vi "GeoData.vi"() -> ()   [LabVIEW 2017] (continued)
H1\n17261\t42055\tSouth mountain\tPA\tFranklin County\tH1\n17225\t42055\tGreencastle\tPA\tFranklin County\tH1\n17257\t42055\tShippensburg\tPA\tFranklin County\tH1\n17263\t42055\tState line\tPA\tFranklin County\tH1\n17251\t42055\tRoxbury\tPA\tFranklin County\tH1\n17211\t42057\tArtemas\tPA\tFulton County\tH1\n17238\t42057\tNeedmore\tPA\tFulton County\tH1\n17228\t42057\tHarrisonville\tPA\tFulton County\tH1\n17264\t42057\tThree springs\tPA\tFulton County\tH1\n17236\t42057\tMercersburg\tPA\tFulton County\tH1\n15533\t42057\tBreezewood\tPA\tFulton County\tH1\n17224\t42057\tFort loudon\tPA\tFulton County\tH1\n16689\t42057\tWaterfall\tPA\tFulton County\tH1\n16691\t42057\tWells tannery\tPA\tFulton County\tH1\n17255\t42057\tShade gap\tPA\tFulton County\tH1\n15536\t42057\tCrystal spring\tPA\tFulton County\tH1\n17233\t42057\tMc connellsburg\tPA\tFulton County\tH1\n17267\t42057\tWarfordsburg\tPA\tFulton County\tH1\n16674\t42057\tRobertsdale\tPA\tFulton County\tH1\n17229\t42057\tHustontown\tPA\tFulton County\tH1\n17212\t42057\tBig cove tannery\tPA\tFulton County\tH1\n17215\t42057\tBurnt cabins\tPA\tFulton County\tH1\n17223\t42057\tFort littleton\tPA\tFulton County\tH1\n15334\t42059\tGarards fort\tPA\tGreene County\tH1\n15461\t42059\tMasontown\tPA\tGreene County\tH1\n15359\t42059\tRogersville\tPA\tGreene County\tH1\n15346\t42059\tMather\tPA\tGreene County\tH1\n15349\t42059\tMount morris\tPA\tGreene County\tH1\n15344\t42059\tJefferson\tPA\tGreene County\tH1\n15315\t42059\tBobtown\tPA\tGreene County\tH1\n15353\t42059\tNineveh\tPA\tGreene County\tH1\n15380\t42059\tWind ridge\tPA\tGreene County\tH1\n15310\t42059\tAleppo\tPA\tGreene County\tH1\n15352\t42059\tNew freeport\tPA\tGreene County\tH1\n15338\t42059\tGreensboro\tPA\tGreene County\tH1\n15320\t42059\tCarmichaels\tPA\tGreene County\tH1\n15329\t42059\tProsperity\tPA\tGreene County\tH1\n15370\t42059\tWaynesburg\tPA\tGreene County\tH1\n15377\t42059\tWest finley\tPA\tGreene County\tH1\n15364\t42059\tSycamore\tPA\tGreene County\tH1\n15325\t42059\tCrucible\tPA\tGreene County\tH1\n15327\t42059\tDilliner\tPA\tGreene County\tH1\n15362\t42059\tSpraggs\tPA\tGreene County\tH1\n15316\t42059\tBrave\tPA\tGreene County\tH1\n15337\t42059\tGraysville\tPA\tGreene County\tH1\n15341\t42059\tHolbrook\tPA\tGreene County\tH1\n15322\t42059\tClarksville\tPA\tGreene County\tH1\n15357\t42059\tRices landing\tPA\tGreene County\tH1\n15351\t42059\tNemacolin\tPA\tGreene County\tH1\n16647\t42061\tHesston\tPA\tHuntingdon County\tH1\n16654\t42061\tHuntingdon\tPA\tHuntingdon County\tH1\n16611\t42061\tAlexandria\tPA\tHuntingdon County\tH1\n16693\t42061\tWilliamsburg\tPA\tHuntingdon County\tH1\n16657\t42061\tJames creek\tPA\tHuntingdon County\tH1\n16865\t42061\tPennsylvania furnace\tPA\tHuntingdon County\tH1\n17066\t42061\tMount union\tPA\tHuntingdon County\tH1\n17264\t42061\tThree springs\tPA\tHuntingdon County\tH1\n16669\t42061\tPetersburg\tPA\tHuntingdon County\tH1\n17021\t42061\tEast waterford\tPA\tHuntingdon County\tH1\n16689\t42061\tWaterfall\tPA\tHuntingdon County\tH1\n17255\t42061\tShade gap\tPA\tHuntingdon County\tH1\n17052\t42061\tMapleton depot\tPA\tHuntingdon County\tH1\n16634\t42061\tDudley\tPA\tHuntingdon County\tH1\n17213\t42061\tBlairs mills\tPA\tHuntingdon County\tH1\n16623\t42061\tCassville\tPA\tHuntingdon County\tH1\n16638\t42061\tEntriken\tPA\tHuntingdon County\tH1\n16685\t42061\tTodd\tPA\tHuntingdon County\tH1\n17060\t42061\tMill creek\tPA\tHuntingdon County\tH1\n17243\t42061\tOrbisonia\tPA\tHuntingdon County\tH1\n16652\t42061\tHuntingdon\tPA\tHuntingdon County\tH1\n16678\t42061\tSaxton\tPA\tHuntingdon County\tH1\n16622\t42061\tCalvin\tPA\tHuntingdon County\tH1\n16683\t42061\tSpruce creek\tPA\tHuntingdon County\tH1\n16686\t42061\tTyrone\tPA\tHuntingdon County\tH1\n16674\t42061\tRobertsdale\tPA\tHuntingdon County\tH1\n17229\t42061\tHustontown\tPA\tHuntingdon County\tH1\n16621\t42061\tBroad top\tPA\tHuntingdon County\tH1\n16877\t42061\tWarriors mark\tPA\tHuntingdon County\tH1\n17002\t42061\tAllensville\tPA\tHuntingdon County\tH1\n17239\t42061\tNeelyton\tPA\tHuntingdon County\tH1\n17249\t42061\tRockhill furnace\tPA\tHuntingdon County\tH1\n16660\t42061\tMc connellstown\tPA\tHuntingdon County\tH1\n17260\t42061\tShirleysburg\tPA\tHuntingdon County\tH1\n17215\t42061\tBurnt cabins\tPA\tHuntingdon County\tH1\n17253\t42061\tSaltillo\tPA\tHuntingdon County\tH1\n16694\t42061\tWood\tPA\tHuntingdon County\tH1\n15734\t42063\tDixonville\tPA\tIndiana County\tH1\n15714\t42063\tNorthern cambria\tPA\tIndiana County\tH1\n15725\t42063\tClarksburg\tPA\tIndiana County\tH1\n15765\t42063\tPenn run\tPA\tIndiana County\tH1\n16222\t42063\tDayton\tPA\tIndiana County\tH1\n15712\t42063\tArcadia\tPA\tIndiana County\tH1\n16246\t42063\tPlumville\tPA\tIndiana County\tH1\n15752\t42063\tKent\tPA\tIndiana County\tH1\n15774\t42063\tShelocta\tPA\tIndiana County\tH1\n16256\t42063\tSmicksburg\tPA\tIndiana County\tH1\n15756\t42063\tMc intyre\tPA\tIndiana County\tH1\n15783\t42063\tWest lebanon\tPA\tIndiana County\tH1\n15745\t42063\tHeilwood\tPA\tIndiana County\tH1\n15731\t42063\tCoral\tPA\tIndiana County\tH1\n15727\t42063\tClune\tPA\tIndiana County\tH1\n15723\t42063\tChambersville\tPA\tIndiana County\tH1\n15618\t42063\tAvonmore\tPA\tIndiana County\tH1\n15701\t42063\tIndiana\tPA\tIndiana County\tH1\n15748\t42063\tHomer city\tPA\tIndiana County\tH1\n15767\t42063\tPunxsutawney\tPA\tIndiana County\tH1\n15957\t42063\tStrongstown\tPA\tIndiana County\tH1\n15949\t42063\tRobinson\tPA\tIndiana County\tH1\n15920\t42063\tArmagh\tPA\tIndiana County\tH1\n15777\t42063\tStarford\tPA\tIndiana County\tH1\n15754\t42063\tLucernemines\tPA\tIndiana County\tH1\n16211\t42063\tBeyer\tPA\tIndiana County\tH1\n15757\t42063\tMahaffey\tPA\tIndiana County\tH1\n15732\t42063\tCreekside\tPA\tIndiana County\tH1\n15759\t42063\tMarion center\tPA\tIndiana County\tH1\n15705\t42063\tIndiana\tPA\tIndiana County\tH1\n15961\t42063\tVintondale\tPA\tIndiana County\tH1\n15684\t42063\tSlickville\tPA\tIndiana County\tH1\n15742\t42063\tGlen campbell\tPA\tIndiana County\tH1\n15724\t42063\tCherry tree\tPA\tIndiana County\tH1\n15747\t42063\tHome\tPA\tIndiana County\tH1\n15713\t42063\tAultman\tPA\tIndiana County\tH1\n15771\t42063\tRochester mills\tPA\tIndiana County\tH1\n15729\t42063\tCommodore\tPA\tIndiana County\tH1\n15758\t42063\tMarchand\tPA\tIndiana County\tH1\n15720\t42063\tBrush valley\tPA\tIndiana County\tH1\n15717\t42063\tBlairsville\tPA\tIndiana County\tH1\n15728\t42063\tClymer\tPA\tIndiana County\tH1\n15681\t42063\tSaltsburg\tPA\tIndiana County\tH1\n15954\t42063\tSeward\tPA\tIndiana County\tH1\n15739\t42063\tErnest\tPA\tIndiana County\tH1\n15716\t42063\tBlack lick\tPA\tIndiana County\tH1\n15746\t42063\tHillsdale\tPA\tIndiana County\tH1\n15750\t42063\tJosephine\tPA\tIndiana County\tH1\n15772\t42063\tRossiter\tPA\tIndiana County\tH1\n15944\t42063\tNew florence\tPA\tIndiana County\tH1\n15761\t42063\tMentcle\tPA\tIndiana County\tH1\n15763\t42063\tNorthpoint\tPA\tIndiana County\tH1\n15929\t42063\tDilltown\tPA\tIndiana County\tH1\n15710\t42063\tAlverda\tPA\tIndiana County\tH1\n15741\t42063\tGipsy\tPA\tIndiana County\tH1\n15801\t42065\tDu bois\tPA\tJefferson County\tH1\n15840\t42065\tFalls creek\tPA\tJefferson County\tH1\n15778\t42065\tTimblin\tPA\tJefferson County\tH1\n15828\t42065\tClarington\tPA\tJefferson County\tH1\n15744\t42065\tHamilton\tPA\tJefferson County\tH1\n15863\t42065\tStump creek\tPA\tJefferson County\tH1\n15730\t42065\tCoolspring\tPA\tJefferson County\tH1\n15853\t42065\tRidgway\tPA\tJefferson County\tH1\n15824\t42065\tBrockway\tPA\tJefferson County\tH1\n15770\t42065\tRinggold\tPA\tJefferson County\tH1\n16222\t42065\tDayton\tPA\tJefferson County\tH1\n15847\t42065\tKnox dale\tPA\tJefferson County\tH1\n15851\t42065\tReynoldsville\tPA\tJefferson County\tH1\n15865\t42065\tSykesville\tPA\tJefferson County\tH1\n15767\t42065\tPunxsutawney\tPA\tJefferson County\tH1\n15829\t42065\tCorsica\tPA\tJefferson County\tH1\n15823\t42065\tBrockport\tPA\tJefferson County\tH1\n15780\t42065\tValier\tPA\tJefferson County\tH1\n15715\t42065\tBig run\tPA\tJefferson County\tH1\n15764\t42065\tOliveburg\tPA\tJefferson County\tH1\n15776\t42065\tSprankle mills\tPA\tJefferson County\tH1\n15711\t42065\tAnita\tPA\tJefferson County\tH1\n15784\t42065\tWorthville\tPA\tJefferson County\tH1\n15733\t42065\tDe lancey\tPA\tJefferson County\tH1\n15781\t42065\tWalston\tPA\tJefferson County\tH1\n16240\t42065\tMayport\tPA\tJefferson County\tH1\n15825\t42065\tBrookville\tPA\tJefferson County\tH1\n15860\t42065\tSigel\tPA\tJefferson County\tH1\n15772\t42065\tRossiter\tPA\tJefferson County\tH1\n15864\t42065\tSummerville\tPA\tJefferson County\tH1\n15763\t42065\tNorthpoint\tPA\tJefferson County\tH1\n17059\t42067\tMifflintown\tPA\tJuniata County\tH1\n17014\t42067\tCocolamus\tPA\tJuniata County\tH1\n17021\t42067\tEast waterford\tPA\tJuniata County\tH1\n17086\t42067\tRichfield\tPA\tJuniata County\tH1\n17049\t42067\tMc alisterville\tPA\tJuniata County\tH1\n17082\t42067\tPort royal\tPA\tJuniata County\tH1\n17094\t42067\tThompsontown\tPA\tJuniata County\tH1\n17035\t42067\tHoney grove\tPA\tJuniata County\tH1\n17056\t42067\tMexico\tPA\tJuniata County\tH1\n17853\t42067\tMount pleasant mills\tPA\tJuniata County\tH1\n17062\t42067\tMillerstown\tPA\tJuniata County\tH1\n17243\t42067\tOrbisonia\tPA\tJuniata County\tH1\n17045\t42067\tLiverpool\tPA\tJuniata County\tH1\n17058\t42067\tMifflin\tPA\tJuniata County\tH1\n17076\t42067\tOakland mills\tPA\tJuniata County\tH1\n18446\t42069\tNicholson\tPA\tLackawanna County\tH1\n18510\t42069\tScranton\tPA\tLackawanna County\tH1\n18505\t42069\tScranton\tPA\tLackawanna County\tH1\n18509\t42069\tScranton\tPA\tLackawanna County\tH1\n18414\t42069\tDalton\tPA\tLackawanna County\tH1\n18444\t42069\tMoscow\tPA\tLackawanna County\tH1\n18504\t42069\tScranton\tPA\tLackawanna County\tH1\n18452\t42069\tPeckville\tPA\tLackawanna County\tH1\n18515\t42069\tScranton\tPA\tLackawanna County\tH1\n18403\t42069\tArchbald\tPA\tLackawanna County\tH1\n18421\t42069\tForest city\tPA\tLackawanna County\tH1\n18518\t42069\tOld forge\tPA\tLackawanna County\tH1\n18503\t42069\tScranton\tPA\tLackawanna County\tH1\n18653\t42069\tRansom\tPA\tLackawanna County\tH1\n18411\t42069\tClarks summit\tPA\tLackawanna County\tH1\n18436\t42069\tLake ariel\tPA\tLackawanna County\tH1\n18472\t42069\tWaymart\tPA\tLackawanna County\tH1\n18512\t42069\tScranton\tPA\tLackawanna County\tH1\n18641\t42069\tPittston\tPA\tLackawanna County\tH1\n18471\t42069\tWaverly\tPA\tLackawanna County\tH1\n18433\t42069\tJermyn\tPA\tLackawanna County\tH1\n18501\t42069\tScranton\tPA\tLackawanna County\tH1\n18420\t42069\tFleetville\tPA\tLackawanna County\tH1\n18519\t42069\tScranton\tPA\tLackawanna County\tH1\n18419\t42069\tFactoryville\tPA\tLackawanna County\tH1\n18434\t42069\tJessup\tPA\tLackawanna County\tH1\n18640\t42069\tPittston\tPA\tLackawanna County\tH1\n18410\t42069\tChinchilla\tPA\tLackawanna County\tH1\n18540\t42069\tScranton\tPA\tLackawanna County\tH1\n18447\t42069\tOlyphant\tPA\tLackawanna County\tH1\n18507\t42069\tMoosic\tPA\tLackawanna County\tH1\n18416\t42069\tElmhurst\tPA\tLackawanna County\tH1\n18440\t42069\tLa plume\tPA\tLackawanna County\tH1\n18448\t42069\tOlyphant\tPA\tLackawanna County\tH1\n18407\t42069\tCarbondale\tPA\tLackawanna County\tH1\n18424\t42069\tGouldsboro\tPA\tLackawanna County\tH1\n18508\t42069\tScranton\tPA\tLackawanna County\tH1\n18517\t42069\tTaylor\tPA\tLackawanna County\tH1\n17033\t42071\tHershey\tPA\tLancaster County\tH1\n17512\t42071\tColumbia\tPA\tLancaster County\tH1\n17535\t42071\tKinzers\tPA\tLancaster County\tH1\n19363\t42071\tOxford\tPA\tLancaster County\tH1\n17520\t42071\tEast petersburg\tPA\tLancaster County\tH1\n17562\t42071\tParadise\tPA\tLancaster County\tH1\n17579\t42071\tStrasburg\tPA\tLancaster County\tH1\n17567\t42071\tReamstown\tPA\tLancaster County\tH1\n17521\t42071\tElm\tPA\tLancaster County\tH1\n17528\t42071\tGoodville\tPA\tLancaster County\tH1\n17585\t42071\tWitmer\tPA\tLancaster County\tH1\n17570\t42071\tRheems\tPA\tLancaster County\tH1\n17501\t42071\tAkron\tPA\tLancaster County\tH1\n17502\t42071\tBainbridge\tPA\tLancaster County\tH1\n17540\t42071\tLeola\tPA\tLancaster County\tH1\n17602\t42071\tLancaster\tPA\tLancaster County\tH1\n17566\t42071\tQuarryville\tPA\tLancaster County\tH1\n19540\t42071\tMohnton\tPA\tLancaster County\tH1\n17532\t42071\tHoltwood\tPA\tLancaster County\tH1\n17536\t42071\tKirkwood\tPA\tLancaster County\tH1\n17604\t42071\tLancaster\tPA\tLancaster County\tH1\n17560\t42071\tNew providence\tPA\tLancaster County\tH1\n17507\t42071\tBowmansville\tPA\tLancaster County\tH1\n17580\t42071\tTalmage\tPA\tLancaster County\tH1\n17503\t42071\tBart\tPA\tLancaster County\tH1\n17552\t42071\tMount joy\tPA\tLancaster County\tH1\n17551\t42071\tMillersville\tPA\tLancaster County\tH1\n17555\t42071\tNarvon\tPA\tLancaster County\tH1\n19543\t42071\tMorgantown\tPA\tLancaster County\tH1\n17581\t42071\tTerre hill\tPA\tLancaster County\tH1\n17699\t42071\tLancaster\tPA\tLancaster County\tH1\n17522\t42071\tEphrata\tPA\tLancaster County\tH1\n17527\t42071\tGap\tPA\tLancaster County\tH1\n17543\t42071\tLititz\tPA\tLancaster County\tH1\n17538\t42071\tLandisville\tPA\tLancaster County\tH1\n17509\t42071\tChristiana\tPA\tLancaster County\tH1\n17603\t42071\tLancaster\tPA\tLancaster County\tH1\n17578\t42071\tStevens\tPA\tLancaster County\tH1\n17564\t42071\tPenryn\tPA\tLancaster County\tH1\n17504\t42071\tBausman\tPA\tLancaster County\tH1\n17575\t42071\tSilver spring\tPA\tLancaster County\tH1\n17550\t42071\tMaytown\tPA\tLancaster County\tH1\n17547\t42071\tMarietta\tPA\tLancaster County\tH1\n17557\t42071\tNew holland\tPA\tLancaster County\tH1\n17582\t42071\tWashington boro\tPA\tLancaster County\tH1\n17572\t42071\tRonks\tPA\tLancaster County\tH1\n19344\t42071\tHoney brook\tPA\tLancaster County\tH1\n17605\t42071\tLancaster\tPA\tLancaster County\tH1\n17534\t42071\tIntercourse\tPA\tLancaster County\tH1\n17533\t42071\tHopeland\tPA\tLancaster County\tH1\n17506\t42071\tBlue ball\tPA\tLancaster County\tH1\n17073\t42071\tNewmanstown\tPA\tLancaster County\tH1\n17529\t42071\tGordonville\tPA\tLancaster County\tH1\n17568\t42071\tRefton\tPA\tLancaster County\tH1\n19551\t42071\tRobesonia\tPA\tLancaster County\tH1\n17518\t42071\tDrumore\tPA\tLancaster County\tH1\n17576\t42071\tSmoketown\tPA\tLancaster County\tH1\n17517\t42071\tDenver\tPA\tLancaster County\tH1\n17608\t42071\tLancaster\tPA\tLancaster County\tH1\n17505\t42071\tBird in hand\tPA\tLancaster County\tH1\n19501\t42071\tAdamstown\tPA\tLancaster County\tH1\n17022\t42071\tElizabethtown\tPA\tLancaster County\tH1\n17314\t42071\tDelta\tPA\tLancaster County\tH1\n17545\t42071\tManheim\tPA\tLancaster County\tH1\n17554\t42071\tMountville\tPA\tLancaster County\tH1\n17519\t42071\tEast earl\tPA\tLancaster County\tH1\n17563\t42071\tPeach bottom\tPA\tLancaster County\tH1\n17601\t42071\tLancaster\tPA\tLancaster County\tH1\n17565\t42071\tPequea\tPA\tLancaster County\tH1\n17569\t42071\tReinholds\tPA\tLancaster County\tH1\n17584\t42071\tWillow street\tPA\tLancaster County\tH1\n19310\t42071\tAtglen\tPA\tLancaster County\tH1\n19362\t42071\tNottingham\tPA\tLancaster County\tH1\n17516\t42071\tConestoga\tPA\tLancaster County\tH1\n17508\t42071\tBrownstown\tPA\tLancaster County\tH1\n17537\t42071\tLampeter\tPA\tLancaster County\tH1\n16051\t42073\tPortersville\tPA\tLawrence County\tH1\n16127\t42073\tGrove city\tPA\tLawrence County\tH1\n16116\t42073\tEdinburg\tPA\tLawrence County\tH1\n16159\t42073\tWest middlesex\tPA\tLawrence County\tH1\n16155\t42073\tVilla maria\tPA\tLawrence County\tH1\n16105\t42073\tNew castle\tPA\tLawrence County\tH1\n16102\t42073\tNew castle\tPA\tLawrence County\tH1\n16601\t42073\tAltoona\tPA\tLawrence County\tH1\n16160\t42073\tWest pittsburg\tPA\tLawrence County\tH1\n16101\t42073\tNew castle\tPA\tLawrence County\tH1\n16120\t42073\tEnon valley\tPA\tLawrence County\tH1\n16117\t42073\tEllwood city\tPA\tLawrence County\tH1\n16112\t42073\tBessemer\tPA\tLawrence County\tH1\n16123\t42073\tFombell\tPA\tLawrence County\tH1\n16142\t42073\tNew wilmington\tPA\tLawrence County\tH1\n16172\t42073\tNew wilmington\tPA\tLawrence County\tH1\n16132\t42073\tHillsville\tPA\tLawrence County\tH1\n16108\t42073\tNew castle\tPA\tLawrence County\tH1\n16157\t42073\tWampum\tPA\tLawrence County\tH1\n16156\t42073\tVolant\tPA\tLawrence County\tH1\n16141\t42073\tNew galilee\tPA\tLawrence County\tH1\n16140\t42073\tNew bedford\tPA\tLawrence County\tH1\n16057\t42073\tSlippery rock\tPA\tLawrence County\tH1\n16037\t42073\tHarmony\tPA\tLawrence County\tH1\n16143\t42073\tPulaski\tPA\tLawrence County\tH1\n17033\t42075\tHershey\tPA\tLebanon County\tH1\n19567\t42075\tWomelsdorf\tPA\tLebanon County\tH1\n17087\t42075\tRichland\tPA\tLebanon County\tH1\n17016\t42075\tCornwall\tPA\tLebanon County\tH1\n17028\t42075\tGrantville\tPA\tLebanon County\tH1\n17046\t42075\tLebanon\tPA\tLebanon County\tH1\n17003\t42075\tAnnville\tPA\tLebanon County\tH1\n17078\t42075\tPalmyra\tPA\tLebanon County\tH1\n17026\t42075\tFredericksburg\tPA\tLebanon County\tH1\n17963\t42075\tPine grove\tPA\tLebanon County\tH1\n17041\t42075\tLawn\tPA\tLebanon County\tH1\n17042\t42075\tLebanon\tPA\tLebanon County\tH1\n17077\t42075\tOno\tPA\tLebanon County\tH1\n17073\t42075\tNewmanstown\tPA\tLebanon County\tH1\n19551\t42075\tRobesonia\tPA\tLebanon County\tH1\n17039\t42075\tKleinfeltersville\tPA\tLebanon County\tH1\n17010\t42075\tCampbelltown\tPA\tLebanon County\tH1\n17064\t42075\tMount gretna\tPA\tLebanon County\tH1\n17083\t42075\tQuentin\tPA\tLebanon County\tH1\n17085\t42075\tRexmont\tPA\tLebanon County\tH1\n17038\t42075\tJonestown\tPA\tLebanon County\tH1\n17067\t42075\tMyerstown\tPA\tLebanon County\tH1\n17545\t42075\tManheim\tPA\tLebanon County\tH1\n17088\t42075\tSchaefferstown\tPA\tLebanon County\tH1\n18032\t42077\tCatasauqua\tPA\tLehigh County\tH1\n18069\t42077\tOrefield\tPA\tLehigh County\tH1\n18066\t42077\tNew tripoli\tPA\tLehigh County\tH1\n18092\t42077\tZionsville\tPA\tLehigh County\tH1\n18080\t42077\tSlatington\tPA\tLehigh County\tH1\n19539\t42077\tMertztown\tPA\tLehigh County\tH1\n18195\t42077\tAllentown\tPA\tLehigh County\tH1\n18068\t42077\tOld zionsville\tPA\tLehigh County\tH1\n18102\t42077\tAllentown\tPA\tLehigh County\tH1\n18106\t42077\tAllentown\tPA\tLehigh County\tH1\n18060\t42077\tLimeport\tPA\tLehigh County\tH1\n18015\t42077\tBethlehem\tPA\tLehigh County\tH1\n18049\t42077\tEmmaus\tPA\tLehigh County\tH1\n18059\t42077\tLaurys station\tPA\tLehigh County\tH1\n19530\t42077\tKutztown\tPA\tLehigh County\tH1\n18951\t42077\tQuakertown\tPA\tLehigh County\tH1\n18087\t42077\tTrexlertown\tPA\tLehigh County\tH1\n18079\t42077\tSlatedale\tPA\tLehigh County\tH1\n18036\t42077\tCoopersburg\tPA\tLehigh County\tH1\n18041\t42077\tEast greenville\tPA\tLehigh County\tH1\n18053\t42077\tGermansville\tPA\tLehigh County\tH1\n18101\t42077\tAllentown\tPA\tLehigh County\tH1\n18105\t42077\tAllentown\tPA\tLehigh County\tH1\n18098\t42077\tEmmaus\tPA\tLehigh County\tH1\n18011\t42077\tAlburtis\tPA\tLehigh County\tH1\n18017\t42077\tBethlehem\tPA\tLehigh County\tH1\n18034\t42077\tCenter valley\tPA\tLehigh County\tH1\n18062\t42077\tMacungie\tPA\tLehigh County\tH1\n18109\t42077\tAllentown\tPA\tLehigh County\tH1\n18052\t42077\tWhitehall\tPA\tLehigh County\tH1\n18104\t42077\tAllentown\tPA\tLehigh County\tH1\n18078\t42077\tSchnecksville\tPA\tLehigh County\tH1\n18046\t42077\tEast texas\tPA\tLehigh County\tH1\n18051\t42077\tFogelsville\tPA\tLehigh County\tH1\n18103\t42077\tAllentown\tPA\tLehigh County\tH1\n18031\t42077\tBreinigsville\tPA\tLehigh County\tH1\n18018\t42077\tBethlehem\tPA\tLehigh County\tH1\n18037\t42077\tCoplay\tPA\tLehigh County\tH1\n19529\t42077\tKempton\tPA\tLehigh County\tH1\n18065\t42077\tNeffs\tPA\tLehigh County\tH1\n18644\t42079\tWyoming\tPA\tLuzerne County\tH1\n18219\t42079\tConyngham\tPA\tLuzerne County\tH1\n18224\t42079\tFreeland\tPA\tLuzerne County\tH1\n18622\t42079\tHuntington mills\tPA\tLuzerne County\tH1\n18711\t42079\tWilkes barre\tPA\tLuzerne County\tH1\n18251\t42079\tSybertsville\tPA\tLuzerne County\tH1\n17814\t42079\tBenton\tPA\tLuzerne County\tH1\n18661\t42079\tWhite haven\tPA\tLuzerne County\tH1\n18655\t42079\tShickshinny\tPA\tLuzerne County\tH1\n18651\t42079\tPlymouth\tPA\tLuzerne County\tH1\n18635\t42079\tNescopeck\tPA\tLuzerne County\tH1\n18634\t42079\tNanticoke\tPA\tLuzerne County\tH1\n18704\t42079\tKingston\tPA\tLuzerne County\tH1\n18706\t42079\tWilkes barre\tPA\tLuzerne County\tH1\n18705\t42079\tWilkes barre\tPA\tLuzerne County\tH1\n17878\t42079\tStillwater\tPA\tLuzerne County\tH1\n18766\t42079\tWilkes barre\tPA\tLuzerne County\tH1\n18602\t42079\tBear creek\tPA\tLuzerne County\tH1\n18762\t42079\tWilkes barre\tPA\tLuzerne County\tH1\n18764\t42079\tWilkes barre\tPA\tLuzerne County\tH1\n18249\t42079\tSugarloaf\tPA\tLuzerne County\tH1\n18222\t42079\tDrums\tPA\tLuzerne County\tH1\n18411\t42079\tClarks summit\tPA\tLuzerne County\tH1\n18618\t42079\tHarveys lake\tPA\tLuzerne County\tH1\n18641\t42079\tPittston\tPA\tLuzerne County\tH1\n18642\t42079\tDuryea\tPA\tLuzerne County\tH1\n18246\t42079\tRock glen\tPA\tLuzerne County\tH1\n18769\t42079\tWilkes barre\tPA\tLuzerne County\tH1\n18225\t42079\tHarleigh\tPA\tLuzerne County\tH1\n17821\t42079\tDanville\tPA\tLuzerne County\tH1\n17815\t42079\tBloomsburg\tPA\tLuzerne County\tH1\n18603\t42079\tBerwick\tPA\tLuzerne County\tH1\n18660\t42079\tWapwallopen\tPA\tLuzerne County\tH1\n18610\t42079\tBlakeslee\tPA\tLuzerne County\tH1\n18621\t42079\tHunlock creek\tPA\tLuzerne County\tH1\n18707\t42079\tMountain top\tPA\tLuzerne County\tH1\n18708\t42079\tShavertown\tPA\tLuzerne County\tH1\n18701\t42079\tWilkes barre\tPA\tLuzerne County\tH1\n18216\t42079\tBeaver meadows\tPA\tLuzerne County\tH1\n18234\t42079\tLattimer mines\tPA\tLuzerne County\tH1\n18239\t42079\tMilnesville\tPA\tLuzerne County\tH1\n18640\t42079\tPittston\tPA\tLuzerne County\tH1\n18657\t42079\tTunkhannock\tPA\tLuzerne County\tH1\n18617\t42079\tGlen lyon\tPA\tLuzerne County\tH1\n18601\t42079\tBeach haven\tPA\tLuzerne County\tH1\n18221\t42079\tDrifton\tPA\tLuzerne County\tH1\n18256\t42079\tWeston\tPA\tLuzerne County\tH1\n18611\t42079\tCambra\tPA\tLuzerne County\tH1\n17985\t42079\tZion grove\tPA\tLuzerne County\tH1\n18201\t42079\tHazleton\tPA\tLuzerne County\tH1\n18255\t42079\tWeatherly\tPA\tLuzerne County\tH1\n18636\t42079\tNoxen\tPA\tLuzerne County\tH1\n18615\t42079\tFalls\tPA\tLuzerne County\tH1\n18656\t42079\tSweet valley\tPA\tLuzerne County\tH1\n18202\t42079\tHazleton\tPA\tLuzerne County\tH1\n18765\t42079\tWilkes barre\tPA\tLuzerne County\tH1\n18223\t42079\tEbervale\tPA\tLuzerne County\tH1\n18627\t42079\tLehman\tPA\tLuzerne County\tH1\n18654\t42079\tShawanese\tPA\tLuzerne County\tH1\n18424\t42079\tGouldsboro\tPA\tLuzerne County\tH1\n18612\t42079\tDallas\tPA\tLuzerne County\tH1\n18643\t42079\tPittston\tPA\tLuzerne County\tH1\n18702\t42079\tWilkes barre\tPA\tLuzerne County\tH1\n18709\t42079\tLuzerne\tPA\tLuzerne County\tH1\n18703\t42079\tWilkes barre\tPA\tLuzerne County\tH1\n18710\t42079\tWilkes barre\tPA\tLuzerne County\tH1\n18247\t42079\tSaint johns\tPA\tLuzerne County\tH1\n17754\t42081\tMontoursville\tPA\tLycoming County\tH1\n17752\t42081\tMontgomery\tPA\tLycoming County\tH1\n16930\t42081\tLiberty\tPA\tLycoming County\tH1\n17763\t42081\tRalston\tPA\tLycoming County\tH1\n17720\t42081\tAntes fort\tPA\tLycoming County\tH1\n17745\t42081\tLock haven\tPA\tLycoming County\tH1\n17703\t42081\tWilliamsport\tPA\tLycoming County\tH1\n17728\t42081\tCogan station\tPA\tLycoming County\tH1\n17771\t42081\tTrout run\tPA\tLycoming County\tH1\n17814\t42081\tBenton\tPA\tLycoming County\tH1\n17765\t42081\tRoaring branch\tPA\tLycoming County\tH1\n17756\t42081\tMuncy\tPA\tLycoming County\tH1\n17702\t42081\tWilliamsport\tPA\tLycoming County\tH1\n17758\t42081\tMuncy valley\tPA\tLycoming County\tH1\n17772\t42081\tTurbotville\tPA\tLycoming County\tH1\n17701\t42081\tWilliamsport\tPA\tLycoming County\tH1\n17723\t42081\tCammal\tPA\tLycoming County\tH1\n17727\t42081\tCedar run\tPA\tLycoming County\tH1\n17705\t42081\tWilliamsport\tPA\tLycoming County\tH1\n17737\t42081\tHughesville\tPA\tLycoming County\tH1\n17810\t42081\tAllenwood\tPA\tLycoming County\tH1\n17776\t42081\tWaterville\tPA\tLycoming County\tH1\n17846\t42081\tMillville\tPA\tLycoming County\tH1\n17739\t42081\tJersey mills\tPA\tLycoming County\tH1\n17742\t42081\tLairdsville\tPA\tLycoming County\tH1\n17762\t42081\tPicture rocks\tPA\tLycoming County\tH1\n16938\t42081\tMorris\tPA\tLycoming County\tH1\n17724\t42081\tCanton\tPA\tLycoming County\tH1\n17747\t42081\tLoganton\tPA\tLycoming County\tH1\n17774\t42081\tUnityville\tPA\tLycoming County\tH1\n17721\t42081\tAvis\tPA\tLycoming County\tH1\n17740\t42081\tJersey shore\tPA\tLycoming County\tH1\n17744\t42081\tLinden\tPA\tLycoming County\tH1\n17769\t42081\tSlate run\tPA\tLycoming County\tH1\n16749\t42083\tSmethport\tPA\tMcKean County\tH1\n16725\t42083\tCuster city\tPA\tMcKean County\tH1\n16745\t42083\tRixford\tPA\tMcKean County\tH1\n15870\t42083\tWilcox\tPA\tMcKean County\tH1\n16701\t42083\tBradford\tPA\tMcKean County\tH1\n16743\t42083\tPort allegany\tPA\tMcKean County\tH1\n16731\t42083\tEldred\tPA\tMcKean County\tH1\n16729\t42083\tDuke center\tPA\tMcKean County\tH1\n16333\t42083\tLudlow\tPA\tMcKean County\tH1\n16732\t42083\tGifford\tPA\tMcKean County\tH1\n16750\t42083\tTurtlepoint\tPA\tMcKean County\tH1\n16726\t42083\tCyclone\tPA\tMcKean County\tH1\n16735\t42083\tKane\tPA\tMcKean County\tH1\n16744\t42083\tRew\tPA\tMcKean County\tH1\n16740\t42083\tMount jewett\tPA\tMcKean County\tH1\n16733\t42083\tHazel hurst\tPA\tMcKean County\tH1\n16748\t42083\tShinglehouse\tPA\tMcKean County\tH1\n16738\t42083\tLewis run\tPA\tMcKean County\tH1\n16730\t42083\tEast smethport\tPA\tMcKean County\tH1\n16724\t42083\tCrosby\tPA\tMcKean County\tH1\n16727\t42083\tDerrick city\tPA\tMcKean County\tH1\n16127\t42085\tGrove city\tPA\tMercer County\tH1\n16159\t42085\tWest middlesex\tPA\tMercer County\tH1\n16134\t42085\tJamestown\tPA\tMercer County\tH1\n16154\t42085\tTransfer\tPA\tMercer County\tH1\n16114\t42085\tClarks mills\tPA\tMercer County\tH1\n16124\t42085\tFredonia\tPA\tMercer County\tH1\n16314\t42085\tCochranton\tPA\tMercer County\tH1\n16038\t42085\tHarrisville\tPA\tMercer County\tH1\n16125\t42085\tGreenville\tPA\tMercer County\tH1\n16121\t42085\tFarrell\tPA\tMercer County\tH1\n16311\t42085\tCarlton\tPA\tMercer County\tH1\n16161\t42085\tWheatland\tPA\tMercer County\tH1\n16151\t42085\tSheakleyville\tPA\tMercer County\tH1\n16113\t42085\tClark\tPA\tMercer County\tH1\n16142\t42085\tNew wilmington\tPA\tMercer County\tH1\n16133\t42085\tJackson center\tPA\tMercer County\tH1\n16137\t42085\tMercer\tPA\tMercer County\tH1\n16148\t42085\tHermitage\tPA\tMercer County\tH1\n16110\t42085\tAdamsville\tPA\tMercer County\tH1\n16146\t42085\tSharon\tPA\tMercer County\tH1\n16130\t42085\tHadley\tPA\tMercer County\tH1\n16156\t42085\tVolant\tPA\tMercer County\tH1\n16150\t42085\tSharpsville\tPA\tMercer County\tH1\n16145\t42085\tSandy lake\tPA\tMercer County\tH1\n16362\t42085\tUtica\tPA\tMercer County\tH1\n16057\t42085\tSlippery rock\tPA\tMercer County\tH1\n16153\t42085\tStoneboro\tPA\tMercer County\tH1\n16143\t42085\tPulaski\tPA\tMercer County\tH1\n16342\t42085\tPolk\tPA\tMercer County\tH1\n17059\t42087\tMifflintown\tPA\tMifflin County\tH1\n17044\t42087\tLewistown\tPA\tMifflin County\tH1\n17004\t42087\tBelleville\tPA\tMifflin County\tH1\n17066\t42087\tMount union\tPA\tMifflin County\tH1\n17054\t42087\tMattawana\tPA\tMifflin County\tH1\n17841\t42087\tMc clure\tPA\tMifflin County\tH1\n17029\t42087\tGranville\tPA\tMifflin County\tH1\n17084\t42087\tReedsville\tPA\tMifflin County\tH1\n17060\t42087\tMill creek\tPA\tMifflin County\tH1\n17009\t42087\tBurnham\tPA\tMifflin County\tH1\n17099\t42087\tYeagertown\tPA\tMifflin County\tH1\n17063\t42087\tMilroy\tPA\tMifflin County\tH1\n17002\t42087\tAllensville\tPA\tMifflin County\tH1\n17075\t42087\tNewton hamilton\tPA\tMifflin County\tH1\n17051\t42087\tMc veytown\tPA\tMifflin County\tH1\n18301\t42089\tEast stroudsburg\tPA\tMonroe County\tH1\n18328\t42089\tDingmans ferry\tPA\tMonroe County\tH1\n18347\t42089\tPocono lake\tPA\tMonroe County\tH1\n18353\t42089\tSaylorsburg\tPA\tMonroe County\tH1\n18342\t42089\tMountainhome\tPA\tMonroe County\tH1\n18332\t42089\tHenryville\tPA\tMonroe County\tH1\n18370\t42089\tSwiftwater\tPA\tMonroe County\tH1\n18372\t42089\tTannersville\tPA\tMonroe County\tH1\n18335\t42089\tMarshalls creek\tPA\tMonroe County\tH1\n18327\t42089\tDelaware water gap\tPA\tMonroe County\tH1\n18302\t42089\tEast stroudsburg\tPA\tMonroe County\tH1\n18321\t42089\tBartonsville\tPA\tMonroe County\tH1\n18325\t42089\tCanadensis\tPA\tMonroe County\tH1\n18350\t42089\tPocono pines\tPA\tMonroe County\tH1\n18354\t42089\tSciota\tPA\tMonroe County\tH1\n18360\t42089\tStroudsburg\tPA\tMonroe County\tH1\n18326\t42089\tCresco\tPA\tMonroe County\tH1\n18344\t42089\tMount pocono\tPA\tMonroe County\tH1\n18466\t42089\tTobyhanna\tPA\tMonroe County\tH1\n18333\t42089\tKresgeville\tPA\tMonroe County\tH1\n18071\t42089\tPalmerton\tPA\tMonroe County\tH1\n18355\t42089\tScotrun\tPA\tMonroe County\tH1\n18346\t42089\tPocono summit\tPA\tMonroe County\tH1\n18610\t42089\tBlakeslee\tPA\tMonroe County\tH1\n18331\t42089\tGilbert\tPA\tMonroe County\tH1\n18357\t42089\tSkytop\tPA\tMonroe County\tH1\n18348\t42089\tPocono lake preserve\tPA\tMonroe County\tH1\n18349\t42089\tPocono manor\tPA\tMonroe County\tH1\n18322\t42089\tBrodheadsville\tPA\tMonroe County\tH1\n18341\t42089\tMinisink hills\tPA\tMonroe County\tH1\n18320\t42089\tAnalomink\tPA\tMonroe County\tH1\n18356\t42089\tShawnee on delaware\tPA\tMonroe County\tH1\n18323\t42089\tBuck hill falls\tPA\tMonroe County\tH1\n18058\t42089\tKunkletown\tPA\tMonroe County\tH1\n18210\t42089\tAlbrightsville\tPA\tMonroe County\tH1\n18324\t42089\tBushkill\tPA\tMonroe County\tH1\n18330\t42089\tEffort\tPA\tMonroe County\tH1\n18334\t42089\tLong pond\tPA\tMonroe County\tH1\n18424\t42089\tGouldsboro\tPA\tMonroe County\tH1\n18352\t42089\tReeders\tPA\tMonroe County\tH1\n19006\t42091\tHuntingdon valley\tPA\tMontgomery County\tH1\n19027\t42091\tElkins park\tPA\tMontgomery County\tH1\n19072\t42091\tNarberth\tPA\tMontgomery County\tH1\n19118\t42091\tPhiladelphia\tPA\tMontgomery County\tH1\n19453\t42091\tMont clare\tPA\tMontgomery County\tH1\n19437\t42091\tGwynedd valley\tPA\tMontgomery County\tH1\n18936\t42091\tMontgomeryville\tPA\tMontgomery County\tH1\n19407\t42091\tAudubon\tPA\tMontgomery County\tH1\n18957\t42091\tSalford\tPA\tMontgomery County\tH1\n19002\t42091\tAmbler\tPA\tMontgomery County\tH1\n19009\t42091\tBryn athyn\tPA\tMontgomery County\tH1\n19031\t42091\tFlourtown\tPA\tMontgomery County\tH1\n19025\t42091\tDresher\tPA\tMontgomery County\tH1\n19083\t42091\tHavertown\tPA\tMontgomery County\tH1\n19115\t42091\tPhiladelphia\tPA\tMontgomery County\tH1\n19468\t42091\tRoyersford\tPA\tMontgomery County\tH1\n19035\t42091\tGladwyne\tPA\tMontgomery County\tH1\n19034\t42091\tFort washington\tPA\tMontgomery County\tH1\n19423\t42091\tCedars\tPA\tMontgomery County\tH1\n19505\t42091\tBechtelsville\tPA\tMontgomery County\tH1\n19512\t42091\tBoyertown\tPA\tMontgomery County\tH1\n18914\t42091\tChalfont\tPA\tMontgomery County\tH1\n18964\t42091\tSouderton\tPA\tMontgomery County\tH1\n19010\t42091\tBryn mawr\tPA\tMontgomery County\tH1\n19044\t42091\tHorsham\tPA\tMontgomery County\tH1\n19438\t42091\tHarleysville\tPA\tMontgomery County\tH1\n19440\t42091\tHatfield\tPA\tMontgomery County\tH1\n19492\t42091\tZieglerville\tPA\tMontgomery County\tH1\n19451\t42091\tMainland\tPA\tMontgomery County\tH1\n19484\t42091\tValley forge\tPA\tMontgomery County\tH1\n18041\t42091\tEast greenville\tPA\tMontgomery County\tH1\n19525\t42091\tGilbertsville\tPA\tMontgomery County\tH1\n19004\t42091\tBala cynwyd\tPA\tMontgomery County\tH1\n19046\t42091\tJenkintown\tPA\tMontgomery County\tH1\n19150\t42091\tPhiladelphia\tPA\tMontgomery County\tH1\n19403\t42091\tNorristown\tPA\tMontgomery County\tH1\n19460\t42091\tPhoenixville\tPA\tMontgomery County\tH1\n19454\t42091\tNorth wales\tPA\tMontgomery County\tH1\n19075\t42091\tOreland\tPA\tMontgomery County\tH1\n19472\t42091\tSassamansville\tPA\tMontgomery County\tH1\n18979\t42091\tWoxall\tPA\tMontgomery County\tH1\n18076\t42091\tRed hill\tPA\tMontgomery County\tH1\n18915\t42091\tColmar\tPA\tMontgomery County\tH1\n19003\t42091\tArdmore\tPA\tMontgomery County\tH1\n19001\t42091\tAbington\tPA\tMontgomery County\tH1\n19053\t42091\tFeasterville trevose\tPA\tMontgomery County\tH1\n19096\t42091\tWynnewood\tPA\tMontgomery County\tH1\n19095\t42091\tWyncote\tPA\tMontgomery County\tH1\n19128\t42091\tPhiladelphia\tPA\tMontgomery County\tH1\n19401\t42091\tNorristown\tPA\tMontgomery County\tH1\n19428\t42091\tConshohocken\tPA\tMontgomery County\tH1\n19462\t42091\tPlymouth meeting\tPA\tMontgomery County\tH1\n19464\t42091\tPottstown\tPA\tMontgomery County\tH1\n19473\t42091\tSchwenksville\tPA\tMontgomery County\tH1\n19474\t42091\tSkippack\tPA\tMontgomery County\tH1\n19477\t42091\tSpring house\tPA\tMontgomery County\tH1\n19490\t42091\tWorcester\tPA\tMontgomery County\tH1\n19435\t42091\tFrederick\tPA\tMontgomery County\tH1\n18958\t42091\tSalfordville\tPA\tMontgomery County\tH1\n19486\t42091\tWest point\tPA\tMontgomery County\tH1\n18971\t42091\tTylersport\tPA\tMontgomery County\tH1\n18054\t42091\tGreen lane\tPA\tMontgomery County\tH1\n18932\t42091\tLine lexington\tPA\tMontgomery County\tH1\n18974\t42091\tWarminster\tPA\tMontgomery County\tH1\n19040\t42091\tHatboro\tPA\tMontgomery County\tH1\n19066\t42091\tMerion station\tPA\tMontgomery County\tH1\n19087\t42091\tWayne\tPA\tMontgomery County\tH1\n19090\t42091\tWillow grove\tPA\tMontgomery County\tH1\n19405\t42091\tBridgeport\tPA\tMontgomery County\tH1\n19422\t42091\tBlue bell\tPA\tMontgomery County\tH1\n19406\t42091\tKing of prussia\tPA\tMontgomery County\tH1\n19443\t42091\tKulpsville\tPA\tMontgomery County\tH1\n19409\t42091\tFairview village\tPA\tMontgomery County\tH1\n18918\t42091\tEarlington\tPA\tMontgomery County\tH1\n19430\t42091\tCreamery\tPA\tMontgomery County\tH1\n18070\t42091\tPalm\tPA\tMontgomery County\tH1\n18073\t42091\tPennsburg\tPA\tMontgomery County\tH1\n19426\t42091\tCollegeville\tPA\tMontgomery County\tH1\n18084\t42091\tSumneytown\tPA\tMontgomery County\tH1\n18074\t42091\tPerkiomenville\tPA\tMontgomery County\tH1\n19504\t42091\tBarto\tPA\tMontgomery County\tH1\n18969\t42091\tTelford\tPA\tMontgomery County\tH1\n19012\t42091\tCheltenham\tPA\tMontgomery County\tH1\n19038\t42091\tGlenside\tPA\tMontgomery County\tH1\n19085\t42091\tVillanova\tPA\tMontgomery County\tH1\n19404\t42091\tNorristown\tPA\tMontgomery County\tH1\n19446\t42091\tLansdale\tPA\tMontgomery County\tH1\n19041\t42091\tHaverford\tPA\tMontgomery County\tH1\n19444\t42091\tLafayette hill\tPA\tMontgomery County\tH1\n19436\t42091\tGwynedd\tPA\tMontgomery County\tH1\n19408\t42091\tEagleville\tPA\tMontgomery County\tH1\n19456\t42091\tOaks\tPA\tMontgomery County\tH1\n19450\t42091\tLederach\tPA\tMontgomery County\tH1\n17756\t42093\tMuncy\tPA\tMontour County\tH1\n17777\t42093\tWatsontown\tPA\tMontour County\tH1\n17772\t42093\tTurbotville\tPA\tMontour County\tH1\n17824\t42093\tElysburg\tPA\tMontour County\tH1\n17821\t42093\tDanville\tPA\tMontour County\tH1\n17815\t42093\tBloomsburg\tPA\tMontour County\tH1\n17847\t42093\tMilton\tPA\tMontour County\tH1\n17820\t42093\tCatawissa\tPA\tMontour County\tH1\n17822\t42093\tDanville\tPA\tMontour County\tH1\n17884\t42093\tWashingtonville\tPA\tMontour County\tH1\n18014\t42095\tBath\tPA\tNorthampton County\tH1\n18032\t42095\tCatasauqua\tPA\tNorthampton County\tH1\n18343\t42095\tMount bethel\tPA\tNorthampton County\tH1\n18015\t42095\tBethlehem\tPA\tNorthampton County\tH1\n18045\t42095\tEaston\tPA\tNorthampton County\tH1\n18064\t42095\tNazareth\tPA\tNorthampton County\tH1\n18067\t42095\tNorthampton\tPA\tNorthampton County\tH1\n18055\t42095\tHellertown\tPA\tNorthampton County\tH1\n18035\t42095\tCherryville\tPA\tNorthampton County\tH1\n18351\t42095\tPortland\tPA\tNorthampton County\tH1\n18085\t42095\tTatamy\tPA\tNorthampton County\tH1\n18077\t42095\tRiegelsville\tPA\tNorthampton County\tH1\n18083\t42095\tStockertown\tPA\tNorthampton County\tH1\n18017\t42095\tBethlehem\tPA\tNorthampton County\tH1\n18040\t42095\tEaston\tPA\tNorthampton County\tH1\n18109\t42095\tAllentown\tPA\tNorthampton County\tH1\n18016\t42095\tBethlehem\tPA\tNorthampton County\tH1\n18002\t42095\tLehigh valley\tPA\tNorthampton County\tH1\n18038\t42095\tDanielsville\tPA\tNorthampton County\tH1\n18063\t42095\tMartins creek\tPA\tNorthampton County\tH1\n18013\t42095\tBangor\tPA\tNorthampton County\tH1\n18042\t42095\tEaston\tPA\tNorthampton County\tH1\n18043\t42095\tEaston\tPA\tNorthampton County\tH1\n18086\t42095\tTreichlers\tPA\tNorthampton County\tH1\n18020\t42095\tBethlehem\tPA\tNorthampton County\tH1\n18018\t42095\tBethlehem\tPA\tNorthampton County\tH1\n18072\t42095\tPen argyl\tPA\tNorthampton County\tH1\n18088\t42095\tWalnutport\tPA\tNorthampton County\tH1\n18091\t42095\tWind gap\tPA\tNorthampton County\tH1\n18044\t42095\tEaston\tPA\tNorthampton County\tH1\n17867\t42097\tRebuck\tPA\tNorthumberland County\tH1\n17868\t42097\tRiverside\tPA\tNorthumberland County\tH1\n17872\t42097\tShamokin\tPA\tNorthumberland County\tH1\n17857\t42097\tNorthumberland\tPA\tNorthumberland County\tH1\n17840\t42097\tLocust gap\tPA\tNorthumberland County\tH1\n17850\t42097\tMontandon\tPA\tNorthumberland County\tH1\n17801\t42097\tSunbury\tPA\tNorthumberland County\tH1\n17866\t42097\tCoal township\tPA\tNorthumberland County\tH1\n17017\t42097\tDalmatia\tPA\tNorthumberland County\tH1\n17756\t42097\tMuncy\tPA\tNorthumberland County\tH1\n17830\t42097\tHerndon\tPA\tNorthumberland County\tH1\n17777\t42097\tWatsontown\tPA\tNorthumberland County\tH1\n17772\t42097\tTurbotville\tPA\tNorthumberland County\tH1\n17824\t42097\tElysburg\tPA\tNorthumberland County\tH1\n17749\t42097\tMc ewensville\tPA\tNorthumberland County\tH1\n17821\t42097\tDanville\tPA\tNorthumberland County\tH1\n17834\t42097\tKulpmont\tPA\tNorthumberland County\tH1\n17847\t42097\tMilton\tPA\tNorthumberland County\tH1\n17820\t42097\tCatawissa\tPA\tNorthumberland County\tH1\n17832\t42097\tMarion heights\tPA\tNorthumberland County\tH1\n17836\t42097\tLeck kill\tPA\tNorthumberland County\tH1\n17730\t42097\tDewart\tPA\tNorthumberland County\tH1\n17823\t42097\tDornsife\tPA\tNorthumberland County\tH1\n17860\t42097\tPaxinos\tPA\tNorthumberland County\tH1\n17941\t42097\tKlingerstown\tPA\tNorthumberland County\tH1\n17865\t42097\tPotts grove\tPA\tNorthumberland County\tH1\n17877\t42097\tSnydertown\tPA\tNorthumberland County\tH1\n17851\t42097\tMount carmel\tPA\tNorthumberland County\tH1\n17881\t42097\tTrevorton\tPA\tNorthumberland County\tH1\n17074\t42099\tNewport\tPA\tPerry County\tH1\n17047\t42099\tLoysville\tPA\tPerry County\tH1\n17090\t42099\tShermans dale\tPA\tPerry County\tH1\n17021\t42099\tEast waterford\tPA\tPerry County\tH1\n17071\t42099\tNew germantown\tPA\tPerry County\tH1\n17069\t42099\tNew buffalo\tPA\tPerry County\tH1\n17035\t42099\tHoney grove\tPA\tPerry County\tH1\n17068\t42099\tNew bloomfield\tPA\tPerry County\tH1\n17053\t42099\tMarysville\tPA\tPerry County\tH1\n17040\t42099\tLandisburg\tPA\tPerry County\tH1\n17062\t42099\tMillerstown\tPA\tPerry County\tH1\n17006\t42099\tBlain\tPA\tPerry County\tH1\n17024\t42099\tElliottsburg\tPA\tPerry County\tH1\n17020\t42099\tDuncannon\tPA\tPerry County\tH1\n17045\t42099\tLiverpool\tPA\tPerry County\tH1\n17037\t42099\tIckesburg\tPA\tPerry County\tH1\n19006\t42101\tHuntingdon valley\tPA\tPhiladelphia County\tH6\n19118\t42101\tPhiladelphia\tPA\tPhiladelphia County\tH6\n19126\t42101\tPhiladelphia\tPA\tPhiladelphia County\tH6\n19141\t42101\tPhiladelphia\tPA\tPhiladelphia County\tH6\n19129\t42101\tPhiladelphia\tPA\tPhiladelphia County\tH6\n19151\t42101\tPhiladelphia\tPA\tPhiladelphia County\tH6\n19147\t42101\tPhiladelphia\tPA\tPhiladelphia County\tH6\n19146\t42101\tPhiladelphia\tPA\tPhiladelphia County\tH6\n19105\t42101\tPhiladelphia\tPA\tPhiladelphia County\tH6\n19109\t42101\tPhiladelphia\tPA\tPhiladelphia County\tH6\n19115\t42101\tPhiladelphia\tPA\tPhiladelphia County\tH6\n19111\t42101\tPhiladelphia\tPA\tPhiladelphia County\tH6\n19116\t42101\tPhiladelphia\tPA\tPhiladelphia County\tH6\n19122\t42101\tPhiladelphia\t
